vi "Calculate_GObject_Rectangle.vi"(8 "error in":errorcluster, 11 "GObject ref":refnum<vi>) -> (0 "error out":errorcluster, 2 "Rectangle":T1, 3 "GObject ref dup":refnum<vi>)   [LabVIEW 2012]
doc: "This VI takes any GObject reference an returns a Rectangle from the position and bounds (width, height) of the object."
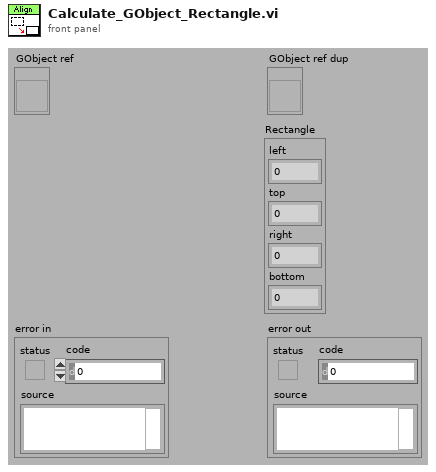
[diagram p1: front panel]
types:
  T1 = cluster{"left":i16, "top":i16, "right":i16, "bottom":i16}
  T2 = typedef "LVPositionTypeDef.ctl" = cluster{"Left":i32, "Top":i32}
  T3 = typedef "LVBoundsTypeDef.ctl" = cluster{"Width":u32, "Height":u32}
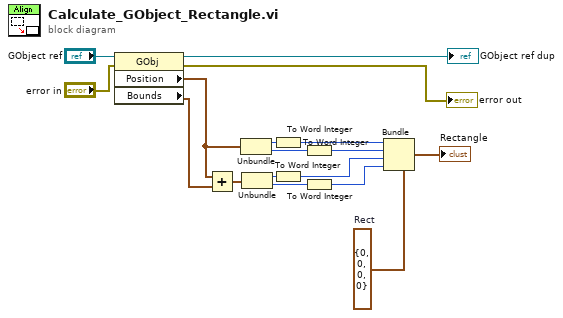
[diagram p0: block diagram]
diagram:
  w17 = T1 {"left"=0, "top"=0, "right"=0, "bottom"=0}  # Rect
  n1 = property class="GObj"(reference="GObject ref", error in="error in") -> (reference out=→"GObject ref dup":refnum<vi>, error out=→"error out":errorcluster, "Position"=w6:T2, "Bounds"=w5:T3)
  n2 = Add(x=w6, y=w5) -> (x+y=w16:T3)
  n3 = Unbundle(w6) -> ("Left"=w14:i32, "Top"=w12:i32)
  n4 = Unbundle(w16) -> ("Width"=w10:u32, "Height"=w9:u32)
  n5 = To Word Integer(number=w14) -> (16bit integer=w13:i16)
  n6 = To Word Integer(number=w10) -> (16bit integer=w8:i16)
  n7 = To Word Integer(number=w12) -> (16bit integer=w11:i16)
  n8 = To Word Integer(number=w9) -> (16bit integer=w7:i16)
  n9 = Bundle(cluster=w17, "left"=w13, "top"=w11, "right"=w8, "bottom"=w7) -> (→"Rectangle":T1)
